vi "Simple_Example_2Cam.vi"() -> ()   [LabVIEW 2019]
doc: "This example shows a simple recording of an image sequence and the image access afterwards for 2 cameras with identical resolution\nIt is a good starting point for writing multi camera applications.\nBut it will not be fail save, i.e. doesnt react on errors, just handles them forward to the end\n\nUsage:\nSelect your required image count before you start the program.\nOnce started, 2 camera classes will be initialized and images will be recorded automatically.\nWhen acquisition has finished you can address the images by index\nTo finish the program click on quit application, this will force fan exit of the camera class"
uses:
  camera/Camera.lvclass
  <vilib>/picture/picture.llb/Draw 8-Bit Pixmap.vi
  <vilib>/picture/picture.llb/Draw True-Color Pixmap.vi
panel:
  in  "Image Index 2":u32 max=9
  out "Recorded Images 2":u32
  out "Image(U16) 2":u16[][](graph)
  out "Image 2":picture
  out "rawImage 2":u16[][](array[numeric])
  out "colormap(U8)":u32[](array[numeric])
  out "Image(U16)":u16[][](graph)
  in  "Zoom [%]":i32(slide)=26 min=10 max=200 step=5 scale=10.0..200.0
  out "Image":picture
  out "rawImage":u16[][](array[numeric])
  in  "data_format":T1(ring)=enum."Mono16"
  in  "Image Index":u32 max=9
  out "Recorded Images":u32
  in  "Quit":bool
  out "Image Height":u16
  out "Image Width":u16
  in  "dwImgCount":u32=10 caption="Required Number of Images" max=4023
  out "Error":errorcluster {"code" format="%x"}
  # "This example shows a simple recording of an image sequence and the image access afterwards for 2 cameras with identical resolution\nIt is a good starting point for writing multi camera applications.\nBut it will not be fail save, i.e. doesnt react on errors, just handles them forward to the end\n\nUsage:\nSelect your required image count before you start the program.\nOnce started, 2 camera classes will be initialized and images will be recorded automatically.\nWhen acquisition has finished you can address the images by index\nTo finish the program click on quit application, this will force fan exit of the camera class"
  # "pco.labview"
  # "Camera Setup"
  # "Recording Control"
  # "Parameters for image readout"
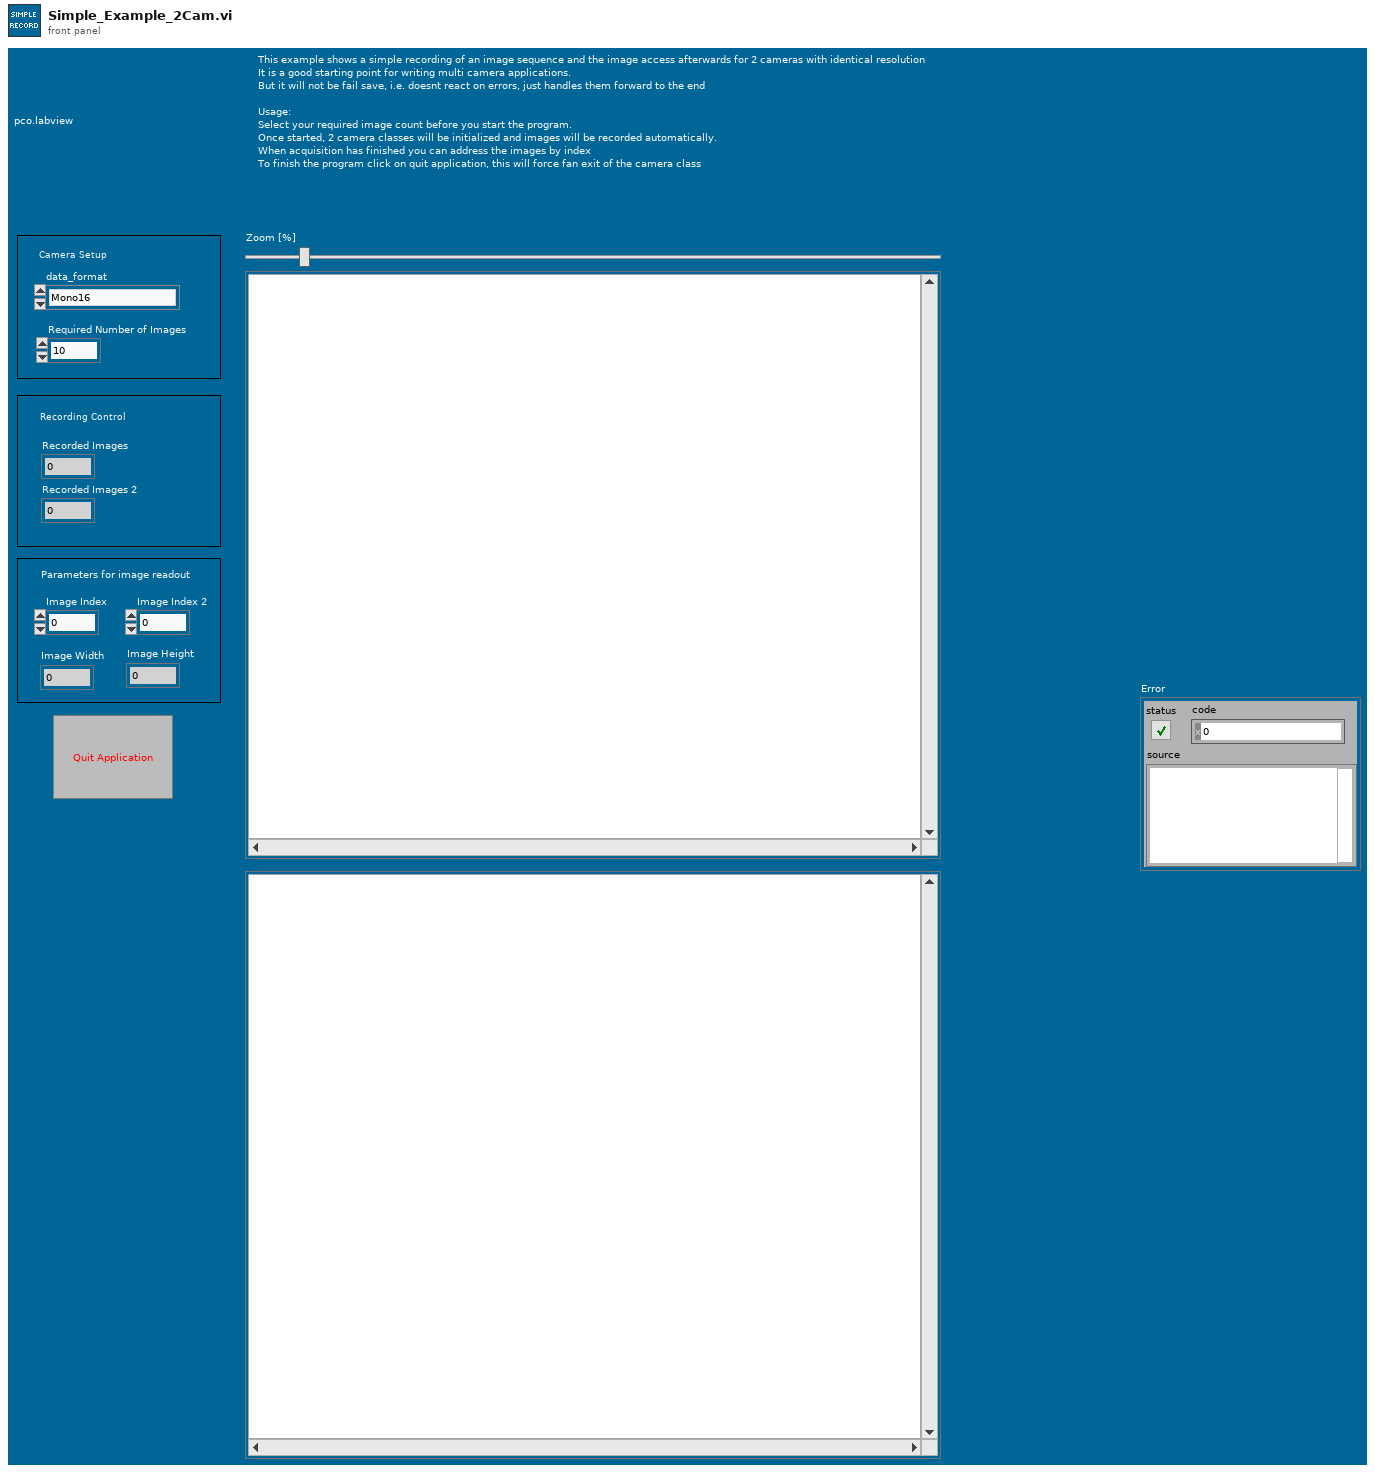
[diagram p1: front panel]
types:
  T1 = enum16{"Undefined", "Mono8", "Mono16", "BGRA8", "RGBA8", "BGRA16", "RGBA16", "CompressedMono8"}
  T2 = enum8{"Enabled", "Disabled", "Disabled and Grayed Out"}
  T3 = enum16{"sequence", "sequence non blocking", "ring buffer", "fifo", "tif", "multitif", "pcoraw", "b16", "dicom", "multidicom", "camram_ring", "camram_segment"}
  T4 = typedef "Camera.lvclass/binning.ctl" = cluster{"vert":u16, "horz":u16, "mode":u16}
  T5 = cluster{"exposure_time_s":dbl, "delay_time_s":dbl, "roi":cluster{"x0":u64, "y0":u64, "x1":u64, "y1":u64}, "timestamp_mode":u16, "pixelrate":u32, "conversion_factor":sgl, "trigger_mode":u16, "acquire_mode":u16, "acquire_sequence_number":u32, "metadata_mode":u16, "noisefilter_mode":u16, "pixel_format":u32, "binning":T4, "auto_exposure":cluster{"region":u16, "min_exposure_s":dbl, "max_exposure_s":dbl}}
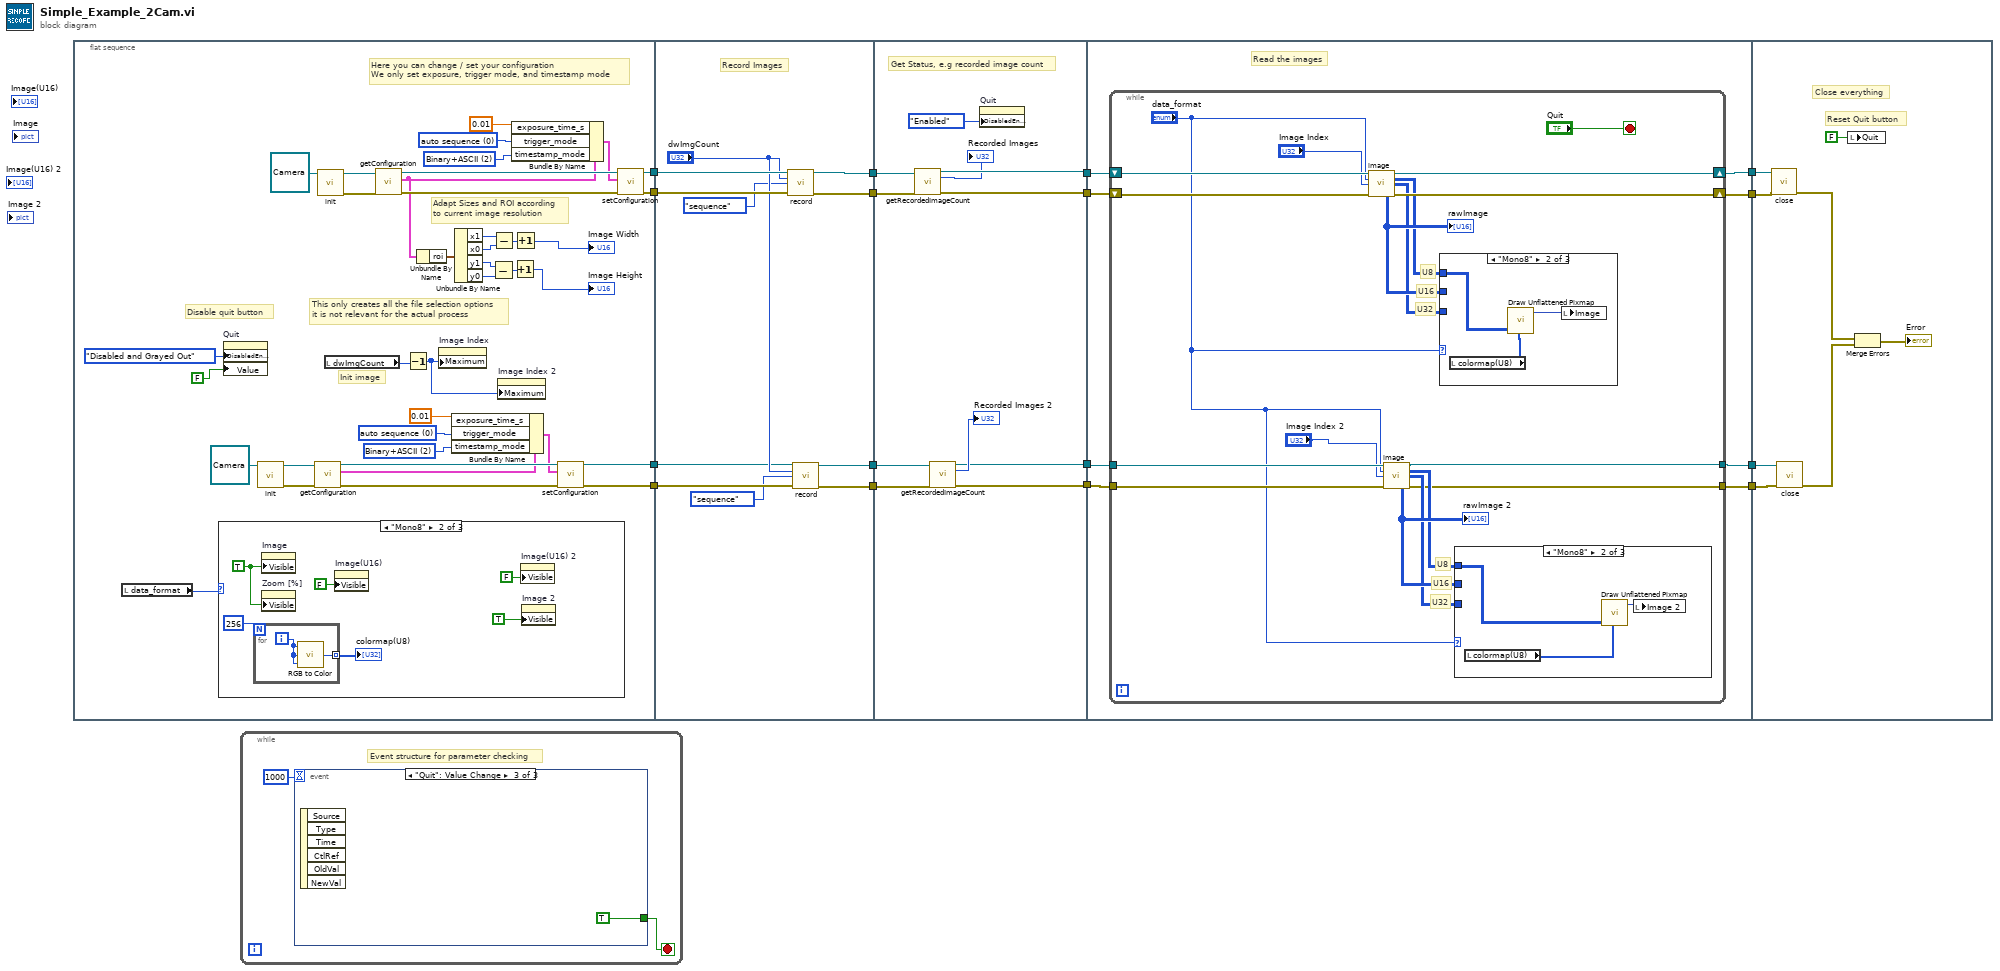
[diagram p0: block diagram]
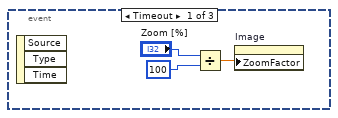
[diagram p2: hidden frame]
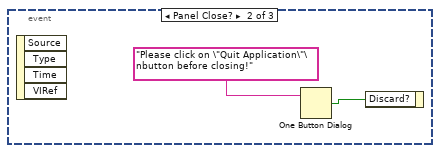
[diagram p3: hidden frame]
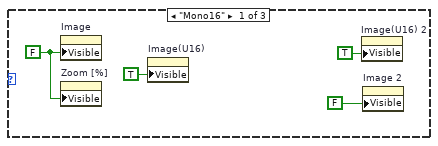
[diagram p4: hidden frame]
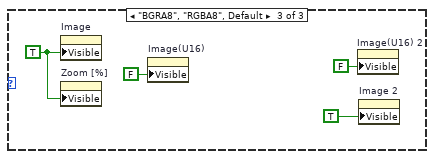
[diagram p5: hidden frame]
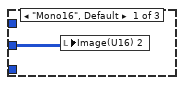
[diagram p6: hidden frame]
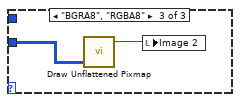
[diagram p7: hidden frame]
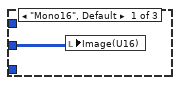
[diagram p8: hidden frame]
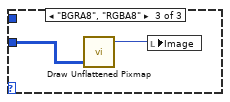
[diagram p9: hidden frame]
diagram:
  n1 = flat-sequence {
    tunnel: [w47] -> w16
    tunnel: [w46] -> w15
    tunnel: [w19] -> w10
    tunnel: [w18] -> w9
    tunnel: w16 -> [w81]
    tunnel: w15 -> [w80]
    tunnel: [w79] -> w14
    tunnel: [w78] -> w13
    tunnel: w10 -> [w76]
    tunnel: w9 -> [w75]
    tunnel: [w74] -> w8
    tunnel: [w73] -> w7
    tunnel: w14 -> [w92]
    tunnel: w13 -> [w91]
    tunnel: [w90] -> w6
    tunnel: [w89] -> w5
    tunnel: w8 -> [w86]
    tunnel: w7 -> [w85]
    tunnel: [w83] -> w4
    tunnel: [w82] -> w3
    tunnel: w6 -> [w99]
    tunnel: w5 -> [w100]
    tunnel: [w98] -> w12
    tunnel: [w97] -> w11
    tunnel: w4 -> [w96]
    tunnel: w3 -> [w95]
    tunnel: [w94] -> w2
    tunnel: [w93] -> w1
    tunnel: w12 -> [w137]
    tunnel: w11 -> [w136]
    tunnel: w2 -> [w132]
    tunnel: w1 -> [w131]
    frame #0 {
      w21 = u16 2 items=["OFF", "Binary", "Binary+ASCII", "ASCII"] ("TimestampMode")
      w26 = u16 0 items=["auto sequence"=0, "software trigger"=1, "external exposure start & software trigger"=2, "external exposure control"=3, "external synchronized"=4, "fast external exposure control"=5, "external CDS control"=6, "slow external exposure control"=7, "external synchronized HDSDI"=258] ("TriggerMode")
      w35 = u16 2 items=["OFF", "Binary", "Binary+ASCII", "ASCII"] ("TimestampMode")
      w51 = u16 0 items=["auto sequence"=0, "software trigger"=1, "external exposure start & software trigger"=2, "external exposure control"=3, "external synchronized"=4, "fast external exposure control"=5, "external CDS control"=6, "slow external exposure control"=7, "external synchronized HDSDI"=258] ("TriggerMode")
      # "Here you can change / set your configuration\nWe only set exposure, trigger mode, and timestamp mode"
      # "Init image"
      # "This only creates all the file selection options\nit is not relevant for the actual process"
      # "Adapt Sizes and ROI according\nto current image resolution"
      # "Disable quit button"
      n2 = local read "data_format"() -> (w31:T1)
      n3 = case shown="\"Mono8\"" w31 {
        frame "Mono16" {
          w58 = FALSE ("Visible")
          n4 = property on="Image" class="Pict"("Visible"=w58) -> ()  [unwired: 2 in, 2 out]
          n5 = property on="Zoom [%]" class="Slide (strict)"("Visible"=w58) -> ()  [unwired: 2 in, 2 out]
          n6 = property on="Image(U16)" class="IntGraph (strict)"("Visible"=TRUE) -> ()  [unwired: 2 in, 2 out]
          n7 = property on="Image(U16) 2" class="IntGraph (strict)"("Visible"=TRUE) -> ()  [unwired: 2 in, 2 out]
          n8 = property on="Image 2" class="Pict"("Visible"=FALSE) -> ()  [unwired: 2 in, 2 out]
        }
        frame "Mono8" {
          w63 = TRUE ("Visible")
          n9 = for {
            N: 256 -> [_]
            tunnel: [w65] -> w62 mode=indexing
            i -> [w66]
            n10 = call <vilib>:"RGB to Color.vi"("B"=w66, "G"=w66, "R"=w66) -> ("Color"=w65:u32)
          }
          "colormap(U8)" <- w62
          n11 = property on="Image" class="Pict"("Visible"=w63) -> ()  [unwired: 2 in, 2 out]
          n12 = property on="Zoom [%]" class="Slide (strict)"("Visible"=w63) -> ()  [unwired: 2 in, 2 out]
          n13 = property on="Image(U16)" class="IntGraph (strict)"("Visible"=FALSE) -> ()  [unwired: 2 in, 2 out]
          n14 = property on="Image(U16) 2" class="IntGraph (strict)"("Visible"=FALSE) -> ()  [unwired: 2 in, 2 out]
          n15 = property on="Image 2" class="Pict"("Visible"=TRUE) -> ()  [unwired: 2 in, 2 out]
        }
        frame "BGRA8", "RGBA8", Default {
          w69 = TRUE ("Visible")
          n16 = property on="Image" class="Pict"("Visible"=w69) -> ()  [unwired: 2 in, 2 out]
          n17 = property on="Zoom [%]" class="Slide (strict)"("Visible"=w69) -> ()  [unwired: 2 in, 2 out]
          n18 = property on="Image(U16)" class="IntGraph (strict)"("Visible"=FALSE) -> ()  [unwired: 2 in, 2 out]
          n19 = property on="Image(U16) 2" class="IntGraph (strict)"("Visible"=FALSE) -> ()  [unwired: 2 in, 2 out]
          n20 = property on="Image 2" class="Pict"("Visible"=TRUE) -> ()  [unwired: 2 in, 2 out]
        }
      }
      n21 = property on="Quit" class="Bool (strict)"("DisabledEnum"=T2."Disabled and Grayed Out" ("Disabled"), "Value"=FALSE ("Stop")) -> ()  [unwired: 2 in, 2 out]
      n22 = call-dynamic "init.vi"("Camera in"=refnum<class "Camera.lvclass"> refnum ("PCOCamera in")) -> ("Camera out"=w28:refnum<class "Camera.lvclass">, "error out"=w27:errorcluster)  [unwired: 8 in]
      n23 = call-dynamic "getConfiguration.vi"("error in (no error)"=w27, "Camera in"=w28) -> ("error out"=w24:errorcluster, "configuration"=w22:T5, "Camera out"=w25:refnum<class "Camera.lvclass">)  [unwired: 7 in]
      n24 = call-dynamic "init.vi"("Camera in"=refnum<class "Camera.lvclass"> refnum ("PCOCamera in")) -> ("Camera out"=w53:refnum<class "Camera.lvclass">, "error out"=w52:errorcluster)  [unwired: 8 in]
      n25 = local read "dwImgCount"() -> (w32:u32)
      n26 = call-dynamic "getConfiguration.vi"("error in (no error)"=w52, "Camera in"=w53) -> ("error out"=w49:errorcluster, "configuration"=w45:T5, "Camera out"=w50:refnum<class "Camera.lvclass">)  [unwired: 7 in]
      n27 = Decrement(x=w32) -> (x-1=w17:u32)
      n28 = Unbundle By Name(w45) -> ("roi"=w44:cluster{"x0":u64, "y0":u64, "x1":u64, "y1":u64})
      n29 = property on="Image Index" class="DigNum (strict)"("Maximum"=w17) -> ()  [unwired: 2 in, 2 out]
      n30 = Bundle By Name(cluster=w22, "exposure_time_s"=0.01, "trigger_mode"=w26, "timestamp_mode"=w21) -> (w23:T5)
      n31 = Unbundle By Name(w44) -> ("x1"=w42:u64, "x0"=w43:u64, "y1"=w40:u64, "y0"=w41:u64)
      n32 = Subtract(x=w40, y=w41) -> (x-y=w38:u64)
      n33 = Subtract(x=w42, y=w43) -> (x-y=w39:u64)
      n34 = property on="Image Index 2" class="DigNum (strict)"("Maximum"=w17) -> ()  [unwired: 2 in, 2 out]
      n35 = Bundle By Name(cluster=w45, "exposure_time_s"=0.01, "trigger_mode"=w51, "timestamp_mode"=w35) -> (w48:T5)
      n36 = Increment(x=w38) -> (x+1=→"Image Height":u64)
      n37 = Increment(x=w39) -> (x+1=→"Image Width":u64)
      n38 = call-dynamic "setConfiguration.vi"("error in (no error)"=w24, "configuration"=w23, "Camera in"=w25) -> ("error out"=w19:errorcluster, "Camera out"=w18:refnum<class "Camera.lvclass">)  [unwired: 7 in]
      n39 = call-dynamic "setConfiguration.vi"("error in (no error)"=w49, "configuration"=w48, "Camera in"=w50) -> ("error out"=w46:errorcluster, "Camera out"=w47:refnum<class "Camera.lvclass">)  [unwired: 7 in]
    }
    frame #1 {
      # "Record Images"
      n40 = call-dynamic "record.vi"("Camera in"=w81, "num_images"="dwImgCount", "record_mode"=T3."sequence", "error in (no error)"=w80) -> ("Camera out"=w79:refnum<class "Camera.lvclass">, "error out"=w78:errorcluster)  [unwired: 10 in]
      n41 = call-dynamic "record.vi"("Camera in"=w75, "num_images"="dwImgCount", "record_mode"=T3."sequence", "error in (no error)"=w76) -> ("Camera out"=w74:refnum<class "Camera.lvclass">, "error out"=w73:errorcluster)  [unwired: 10 in]
    }
    frame #2 {
      # "Get Status, e.g recorded image count"
      n42 = call-dynamic "getRecordedImageCount.vi"("Camera in"=w92, "error in (no error)"=w91) -> ("Camera out"=w90:refnum<class "Camera.lvclass">, "recorded_image_count"=→"Recorded Images":u32, "error out"=w89:errorcluster)  [unwired: 11 in]
      n43 = call-dynamic "getRecordedImageCount.vi"("Camera in"=w86, "error in (no error)"=w85) -> ("Camera out"=w83:refnum<class "Camera.lvclass">, "recorded_image_count"=→"Recorded Images 2":u32, "error out"=w82:errorcluster)  [unwired: 11 in]
      n44 = property on="Quit" class="Bool (strict)"("DisabledEnum"=T2."Enabled" ("Disabled")) -> ()  [unwired: 2 in, 2 out]
    }
    frame #3 {
      # "Read the images"
      n45 = while {
        shift-right: [w116] -> w98
        shift-left: w99 -> [w118]
        shift-right: [w115] -> w97
        shift-left: w100 -> [w117]
        tunnel: w96 -> [w106]
        tunnel: w95 -> [w105]
        tunnel: [w104] -> w94
        tunnel: [w103] -> w93
        stop <- "Quit" stop-if-true
        # "U32"
        # "U16"
        # "U8"
        # "U32"
        # "U16"
        # "U8"
        n46 = call-dynamic "image.vi"("Camera in"=w118, "data_format"="data_format", "image_index"="Image Index", "error in (no error)"=w117) -> ("Camera out"=w116:refnum<class "Camera.lvclass">, "image (U8)"=w110:u8[][], "image (U32)"=w111:u32[][], "raw_image (U16)"=w112:u16[][], "error out"=w115:errorcluster)  [unwired: 3 in, 4 out]
        "rawImage" <- w112
        n47 = call-dynamic "image.vi"("Camera in"=w106, "data_format"="data_format", "image_index"="Image Index 2", "error in (no error)"=w105) -> ("Camera out"=w104:refnum<class "Camera.lvclass">, "image (U8)"=w107:u8[][], "image (U32)"=w108:u32[][], "raw_image (U16)"=w109:u16[][], "error out"=w103:errorcluster)  [unwired: 3 in, 4 out]
        "rawImage 2" <- w109
        n48 = case shown="\"Mono8\"" "data_format" {
          tunnel: w111 -> [_ _ w130]
          tunnel: w110 -> [_ w127 _]
          tunnel: w112 -> [w125 _ _]
          frame "Mono16", Default {
            n49 = local write "Image(U16)"(w125) -> ()
          }
          frame "Mono8" {
            n50 = local read "colormap(U8)"() -> (w126:u32[])
            n51 = call-poly <vilib>:"Draw Unflattened Pixmap.vi"("data"=w127, "color table"=w126) -> ("new picture"=w128:picture)  [unwired: 7 in]
            n52 = local write "Image"(w128) -> ()
          }
          frame "BGRA8", "RGBA8" {
            n53 = call-poly <vilib>:"Draw Unflattened Pixmap.vi"("data (RGB format)"=w130) -> ("new picture"=w129:picture)  [unwired: 8 in]
            n54 = local write "Image"(w129) -> ()
          }
        }
        n55 = case shown="\"Mono8\"" "data_format" {
          tunnel: w108 -> [_ _ w124]
          tunnel: w107 -> [_ w121 _]
          tunnel: w109 -> [w119 _ _]
          frame "Mono16", Default {
            n56 = local write "Image(U16) 2"(w119) -> ()
          }
          frame "Mono8" {
            n57 = local read "colormap(U8)"() -> (w120:u32[])
            n58 = call-poly <vilib>:"Draw Unflattened Pixmap.vi"("data"=w121, "color table"=w120) -> ("new picture"=w122:picture)  [unwired: 7 in]
            n59 = local write "Image 2"(w122) -> ()
          }
          frame "BGRA8", "RGBA8" {
            n60 = call-poly <vilib>:"Draw Unflattened Pixmap.vi"("data (RGB format)"=w124) -> ("new picture"=w123:picture)  [unwired: 8 in]
            n61 = local write "Image 2"(w123) -> ()
          }
        }
      }
    }
    frame #4 {
      # "Reset Quit button"
      # "Close everything"
      n62 = call-dynamic "close.vi"("error in (no error)"=w136, "Camera in"=w137) -> ("error out"=w135:errorcluster)  [unwired: 9 in]
      n63 = call-dynamic "close.vi"("error in (no error)"=w131, "Camera in"=w132) -> ("error out"=w134:errorcluster)  [unwired: 9 in]
      n64 = local write "Quit"(FALSE ("Stop")) -> ()
      n65 = Merge Errors(w135, w134) -> (→"Error":errorcluster)
    }
  }
  n66 = while {
    stop <- w139 stop-if-true
    # "Event structure for parameter checking"
    n67 = event shown="[2] \"Quit\": Value Change" {
      selector: _ -> [_ _ _]
      dyn-events: _ -> [_ _ _]
      timeout: 1000 -> [_ _ _]
      tunnel: [_ _ TRUE] -> w139
      event Timeout {
        n68 = event-data() -> ()  [unwired: 1 in, 3 out]
        n69 = Divide(x="Zoom [%]", y=100 ("Zoom [%]")) -> (x/y=w141:dbl)
        n70 = property on="Image" class="Pict"("ZoomFactor"=w141) -> ()  [unwired: 2 in, 2 out]
      }
      event Panel Close? {
        n71 = event-data() -> ()  [unwired: 1 in, 4 out]
        n72 = One Button Dialog(message="Please click on \"Quit Application\"\nbutton before closing!") -> (true=w144:bool)  [unwired: 1 in]
        n73 = event-data("Discard?"=w144) -> ()  [unwired: 1 in, 1 out]
      }
      event "Quit": Value Change {
        n74 = event-data() -> ()  [unwired: 1 in, 6 out]
      }
    }
  }
